vi "Query Sys (To) Parameters.vi"   [LabVIEW 2012, in "Quantum Composers 9000 Series.lvlib"]
doc: "This polymorphic VI contains VIs to read the mode configuration of the system timer (To)."
uses:
  Quantum Composers 9000 Series.lvlib
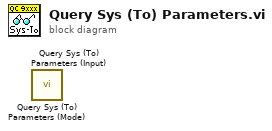
[diagram p0: block diagram]
diagram:
  n1 = call "Query Sys (To) Parameters (Mode).vi"() -> ()  [unwired: 9 in, 3 out]
  n2 = call "Query Sys (To) Parameters (Input).vi"() -> ()  [unwired: 9 in, 3 out]
